vi "form_field.vi"(6 "Template Field Type":T1, 7 "Name":string, 8 "Override data value":bool, 9 "Value":variant, 10 "Form Data":T2[](array[typedef]), 11 "Template Fields":T3[](array[typedef])) -> (1 "field value":string, 2 "Form Data":T2[](array[typedef]), 3 "Template Fields":T3[](array[typedef]))   [LabVIEW 2011]
uses:
  html_form_field.ctl
  template_field.ctl
  template_field_type.ctl
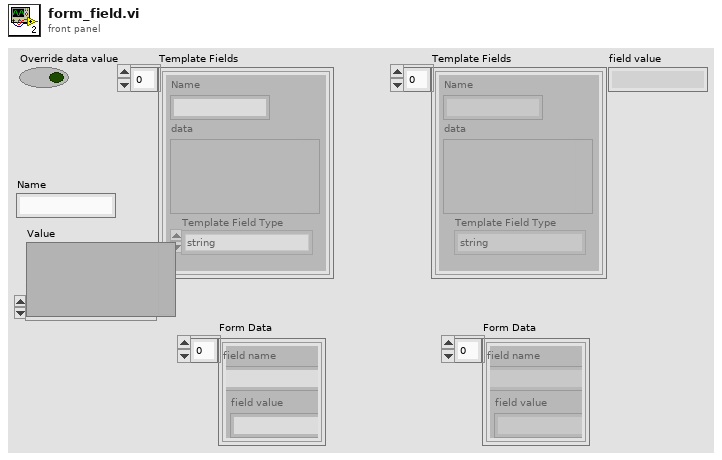
[diagram p1: front panel]
types:
  T1 = typedef "template_field_type.ctl" = enum16{"string", "string array", "number", "number array", "cluster", "cluster array"}
  T2 = typedef "html_form_field.ctl" = cluster{"field name":string, "field value":string}
  T3 = typedef "template_field.ctl" = cluster{"Name":string, "Template Field Type":T1, "data":variant}
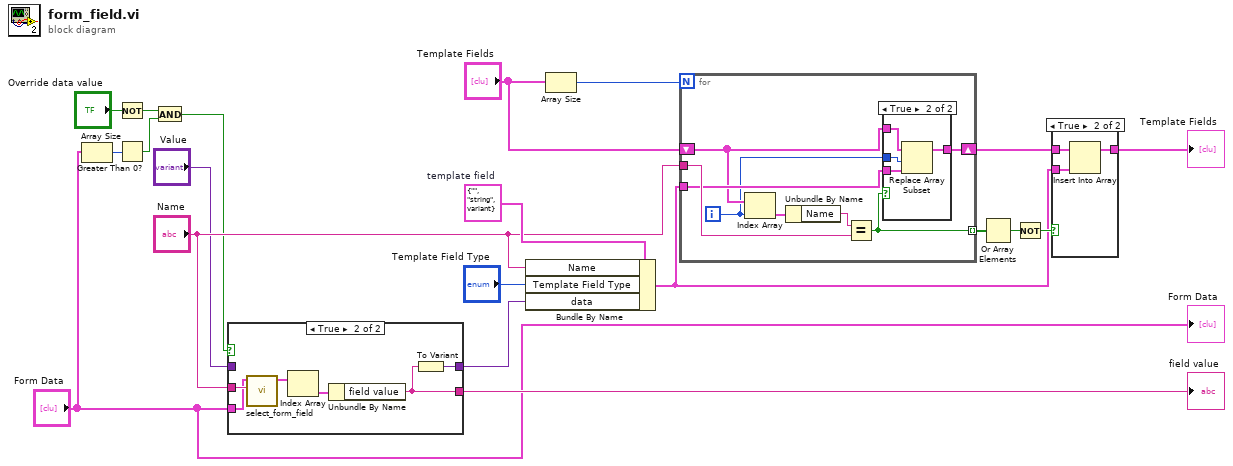
[diagram p0: block diagram]
diagram:
  w18 = T3 {"Name"="", "Template Field Type"=enum."string", "data"=variant}  # template field
  n1 = Array Size(array="Form Data") -> (size(s)=w7:i32)
  n2 = Not(x="Override data value") -> (.not. x?=w1:bool)
  n3 = Greater Than 0?(x=w7) -> (x > 0?=w6:bool)
  n4 = And(x=w1, y=w6) -> (x .and. y?=w3:bool)
  n5 = case shown="True" w3 {
    tunnel: [_ w23] -> w20
    tunnel: "Name" -> [_ w25]
    tunnel: "Form Data" -> [_ w24]
    tunnel: [w21 w22] -> w5
    tunnel: "Value" -> [w21 _]
    frame False {
    }
    frame True {
      n6 = call "select_form_field.vi"("Name"=w25, "Form Data"=w24) -> ("Form Data"=w27:T2[])  [unwired: 8 in, 1 out]
      n7 = Index Array(array=w27) -> (element=w26:T2)  [unwired: 1 in]
      n8 = Unbundle By Name(w26) -> ("field value"=w23:string)
      n9 = To Variant(anything=w23) -> (Variant=w22:variant)
    }
  }
  "field value" <- w20
  n10 = Bundle By Name(cluster=w18, "Name"="Name", "Template Field Type"="Template Field Type", "data"=w5) -> (w12:T3)
  n11 = Array Size(array="Template Fields") -> (size(s)=w10:i32)
  n12 = for {
    N: w10 -> [_]
    tunnel: "Name" -> [w34]
    tunnel: w12 -> [w33]
    shift-right: [w30] -> w13
    shift-left: "Template Fields" -> [w31]
    tunnel: [w28] -> w16 mode=indexing
    i -> [w29]
    n13 = Index Array(array=w31, index=w29) -> (element=w32:T3)
    n14 = Unbundle By Name(w32) -> ("Name"=w35:string)
    n15 = Equal?(x=w35, y=w34) -> (x = y?=w28:bool)
    n16 = case shown="True" w28 {
      tunnel: w33 -> [_ w38]
      tunnel: w31 -> [w36 w40]
      tunnel: [w36 w39] -> w30
      tunnel: w29 -> [_ w37]
      frame False {
      }
      frame True {
        n17 = Replace Array Subset(array=w40, new element=w38, index=w37) -> (w39:T3[])
      }
    }
  }
  n18 = Or Array Elements(Boolean array=w16) -> (logical OR=w15:bool)
  n19 = Not(x=w15) -> (.not. x?=w14:bool)
  n20 = case shown="True" w14 {
    tunnel: w13 -> [w41 w43]
    tunnel: [w41 w44] -> w11
    tunnel: w12 -> [_ w42]
    frame False {
    }
    frame True {
      n21 = Insert Into Array(array=w43, new element=w42) -> (w44:T3[])  [unwired: 1 in]
    }
  }
  "Template Fields" <- w11
  "Form Data" <- "Form Data"
